vi "S4GUI.vi"(7 "Tab ObsEng":enum32{"Obs", "CCD modes", "Eng"}(tab)) -> ()   [LabVIEW 2018] (continued)
                n2773 = call "Write flatted cluster.vi"("error in (no error)"=w6126, "flatted cluster"=w6127, "Interface in"=w6081) -> ("error out"=w6123:errorcluster, "Interface out"=w6124:refnum<class "Interface.lvclass">)  [unwired: 7 in]
                n2774 = call-dynamic "Write Interface.vi"("error in (no error)"=w6123, "Interface.lvclass"=w6124, "Channel in"=w6076) -> ("error out"=w6121:errorcluster, "Channel out"=w6120:refnum<class "Channel.lvclass">)  [unwired: 7 in]
                n2775 = call "Write section_name.vi"("error in (no error)"=w6121, "section_name"="CCD_ACS4", "Channel in"=w6120) -> ("error out"=w6122:errorcluster, "Channel out"=w6117:refnum<class "Channel.lvclass">)  [unwired: 7 in]
                n2776 = call-dynamic "save config.vi"("error in (no error)"=w6122, "file config"="lastsaved.cfg", "Channel in"=w6117) -> ("error out"=w6099:errorcluster, "Channel out"=w6101:refnum<class "Channel.lvclass">)  [unwired: 7 in]
                n2777 = local read "Filter4"() -> (w6098:u8)
                n2778 = call-dynamic "Write Filter.vi"("error in (no error)"=w6099, "Filter"=w6098, "Channel in"=w6101) -> ("error out"=w6112:errorcluster, "Channel out"=w6100:refnum<class "Channel.lvclass">)  [unwired: 7 in]
                n2779 = call-dynamic "Read Interface.vi"("error in (no error)"=w6112, "Channel in"=w6100) -> ("error out"=w6111:errorcluster, "Interface.lvclass"=w6110:refnum<class "Interface.lvclass">, "Channel out"=w6052:refnum<class "Channel.lvclass">)  [unwired: 7 in]
                n2780 = call-dynamic "Write Suffix.vi"("error in (no error)"=w6111, "Suffix"=w6091, "Interface in"=w6110) -> ("error out"=w6102:errorcluster, "Interface out"=w6105:refnum<class "Interface.lvclass">)  [unwired: 7 in]
                n2781 = call-dynamic "Write ObsType.vi"("error in (no error)"=w6102, "ObsType"=w6090, "Interface in"=w6105) -> ("error out"=w6103:errorcluster, "Interface out"=w6106:refnum<class "Interface.lvclass">)  [unwired: 7 in]
                n2782 = call-dynamic "Write Object.vi"("error in (no error)"=w6103, "Object"=w6097, "Interface in"=w6106) -> ("error out"=w6104:errorcluster, "Interface out"=w6107:refnum<class "Interface.lvclass">)  [unwired: 7 in]
                n2783 = call-dynamic "Write Comments.vi"("error in (no error)"=w6104, "Comments"=w6096, "Interface in"=w6107) -> ("error out"=w6108:errorcluster, "Interface out"=w6109:refnum<class "Interface.lvclass">)  [unwired: 7 in]
                n2784 = call-dynamic "Write Observer.vi"("error in (no error)"=w6108, "Observer"=w6095, "Interface in"=w6109) -> ("error out"=w6050:errorcluster, "Interface out"=w6051:refnum<class "Interface.lvclass">)  [unwired: 7 in]
                n2785 = call-dynamic "Write Interface.vi"("error in (no error)"=w6050, "Interface.lvclass"=w6051, "Channel in"=w6052) -> ("error out"=w6059:errorcluster, "Channel out"=w6060:refnum<class "Channel.lvclass">)  [unwired: 7 in]
                n2786 = call-dynamic "Read State Machine.vi"("error in (no error)"=w6059, "Device in"=w6060) -> ("error out"=w6073:errorcluster, "State Machine.lvclass"=w6056:refnum<class "State Machine.lvclass">, "Device out"=w6061:refnum<class "Channel.lvclass">)  [unwired: 7 in]
                n2787 = call-dynamic "Read ref StatesQueue.vi"("error in (no error)"=w6073, "State Machine in"=w6056) -> ("error out"=w6071:errorcluster, "ref StatesQueue"=w6072:refnum<queue>, "State Machine out"=w6055:refnum<class "State Machine.lvclass">)  [unwired: 7 in]
                n2788 = Flush Queue(queue=w6072, error in (no error)=w6071) -> (queue out=w6070:refnum<queue>, error out=w6066:errorcluster)  [unwired: 1 out]
                n2789 = Enqueue Element(queue=w6070, element=u32 300 ("State"), error in (no error)=w6066) -> (queue out=w6069:refnum<queue>, error out=w6065:errorcluster)  [unwired: 1 in, 1 out]
                n2790 = Enqueue Element(queue=w6069, element=u32 60 ("State"), error in (no error)=w6065) -> (queue out=w6068:refnum<queue>, error out=w6067:errorcluster)  [unwired: 1 in, 1 out]
                n2791 = call-dynamic "Write ref StatesQueue.vi"("error in (no error)"=w6067, "ref StatesQueue"=w6068, "State Machine in"=w6055) -> ("error out"=w6064:errorcluster, "State Machine out"=w6054:refnum<class "State Machine.lvclass">)  [unwired: 7 in]
                n2792 = call-dynamic "Write State.vi"("error in (no error)"=w6064, "State"=0, "State Machine in"=w6054) -> ("error out"=w6075:errorcluster, "State Machine out"=w6053:refnum<class "State Machine.lvclass">)  [unwired: 7 in]
                n2793 = call-dynamic "Write State Machine.vi"("error in (no error)"=w6075, "State Machine.lvclass"=w6053, "Device in"=w6061) -> ("error out"=w6058:errorcluster, "Device out"=w6057:refnum<class "Channel.lvclass">)  [unwired: 7 in]
                n2794 = call-dynamic "Write Channel.vi"("error in (no error)"=w6058, "Channel.lvclass"=w6057, "Acquisition in"=w6130) -> ("error out"=w6113:errorcluster, "Acquisition out"=w6114:refnum<class "Acquisition.lvclass">)  [unwired: 7 in]
              }
            }
            n2795 = case shown="True" w6035 {
              tunnel: [w6327 w6406] -> w6046
              tunnel: [w6328 w6405] -> w6047
              tunnel: w6037 -> [w6328 w6388]
              tunnel: w6036 -> [w6327 w6387]
              tunnel: w6019 -> [_ w6366]
              tunnel: w6018 -> [_ w6365]
              tunnel: w6017 -> [_ w6364]
              tunnel: w6016 -> [_ w6360]
              tunnel: w6015 -> [_ w6359]
              frame False {
              }
              frame True {
                # "nome do arquivo .cfg"
                # "seção no arquivo .cfg"
                # "open"
                n2796 = call-dynamic "Read Channel.vi"("error in (no error)"=w6387, "Acquisition in"=w6388) -> ("error out"=w6407:errorcluster, "Channel.lvclass"=w6408:refnum<class "Channel.lvclass">, "Acquisition out"=w6409:refnum<class "Acquisition.lvclass">)  [unwired: 7 in]
                n2797 = call-dynamic "Read Interface.vi"("error in (no error)"=w6407, "Channel in"=w6408) -> ("error out"=w6357:errorcluster, "Interface.lvclass"=w6358:refnum<class "Interface.lvclass">, "Channel out"=w6347:refnum<class "Channel.lvclass">)  [unwired: 7 in]
                n2798 = call-dynamic "Read restoreExpTime.vi"("error in (no error)"=w6357, "Interface in"=w6358) -> ("error out"=w6355:errorcluster, "restoreExpTime"=w6354:bool, "Interface out"=w6356:refnum<class "Interface.lvclass">)  [unwired: 7 in]
                n2799 = case shown="True" w6354 {
                  tunnel: w6356 -> [w6411 w6416]
                  tunnel: [w6411 w6419] -> w6362
                  tunnel: w6355 -> [w6410 w6414]
                  tunnel: [w6410 w6418] -> w6361
                  frame False {
                  }
                  frame True {
                    n2800 = call-dynamic "Write restoreExpTime.vi"("error in (no error)"=w6414, "restoreExpTime"=FALSE, "Interface in"=w6416) -> ("error out"=w6413:errorcluster, "Interface out"=w6415:refnum<class "Interface.lvclass">)  [unwired: 7 in]
                    n2801 = call-dynamic "Read prev ExpTime.vi"("error in (no error)"=w6413, "Interface in"=w6415) -> ("error out"=w6418:errorcluster, "prev ExpTime"=w6417:dbl, "Interface out"=w6419:refnum<class "Interface.lvclass">)  [unwired: 7 in]
                    n2802 = property on="Exptime ch1" class="DigNum (strict)"("Value"=w6417) -> ()  [unwired: 2 in, 2 out]
                  }
                }
                n2803 = call-dynamic "Read PREV_FT.vi"("error in (no error)"=w6361, "Interface in"=w6362) -> ("error out"=w6353:errorcluster, "PREV_FT"=w6363:bool, "Interface out"=w6352:refnum<class "Interface.lvclass">)  [unwired: 7 in]
                n2804 = call-dynamic "Read target cluster.vi"("error in (no error)"=w6353, "Channel in"=w6347) -> ("error out"=w6348:errorcluster, "target cluster"=w6351:T30, "Channel out"=w6346:refnum<class "Channel.lvclass">)  [unwired: 7 in]
                n2805 = Bundle By Name(cluster=w6351, "SHUTTER_MODE"=u8 1, "FRAME_TRANSFER"=w6363) -> (w6350:T30)
                n2806 = call-dynamic "Write target cluster.vi"("error in (no error)"=w6348, "target cluster"=w6350, "Channel in"=w6346) -> ("error out"=w6349:errorcluster, "Channel out"=w6345:refnum<class "Channel.lvclass">)  [unwired: 7 in]
                n2807 = Flatten To String(anything=w6350, error in (no error)=w6349) -> (data string=w6404:string, error out=w6403:errorcluster)  [unwired: 2 in, 1 out]
                n2808 = call "Write flatted cluster.vi"("error in (no error)"=w6403, "flatted cluster"=w6404, "Interface in"=w6352) -> ("error out"=w6400:errorcluster, "Interface out"=w6401:refnum<class "Interface.lvclass">)  [unwired: 7 in]
                n2809 = call-dynamic "Write Interface.vi"("error in (no error)"=w6400, "Interface.lvclass"=w6401, "Channel in"=w6345) -> ("error out"=w6397:errorcluster, "Channel out"=w6396:refnum<class "Channel.lvclass">)  [unwired: 7 in]
                n2810 = call "Write section_name.vi"("error in (no error)"=w6397, "section_name"="CCD_ACS1", "Channel in"=w6396) -> ("error out"=w6398:errorcluster, "Channel out"=w6393:refnum<class "Channel.lvclass">)  [unwired: 7 in]
                n2811 = call-dynamic "save config.vi"("error in (no error)"=w6398, "file config"="lastsaved.cfg", "Channel in"=w6393) -> ("error out"=w6370:errorcluster, "Channel out"=w6369:refnum<class "Channel.lvclass">)  [unwired: 7 in]
                n2812 = local read "Filter1"() -> (w6371:u8)
                n2813 = call-dynamic "Write Filter.vi"("error in (no error)"=w6370, "Filter"=w6371, "Channel in"=w6369) -> ("error out"=w6386:errorcluster, "Channel out"=w6385:refnum<class "Channel.lvclass">)  [unwired: 7 in]
                n2814 = call-dynamic "Read Interface.vi"("error in (no error)"=w6386, "Channel in"=w6385) -> ("error out"=w6382:errorcluster, "Interface.lvclass"=w6381:refnum<class "Interface.lvclass">, "Channel out"=w6375:refnum<class "Channel.lvclass">)  [unwired: 7 in]
                n2815 = call-dynamic "Write Suffix.vi"("error in (no error)"=w6382, "Suffix"=w6360, "Interface in"=w6381) -> ("error out"=w6372:errorcluster, "Interface out"=w6376:refnum<class "Interface.lvclass">)  [unwired: 7 in]
                n2816 = call-dynamic "Write ObsType.vi"("error in (no error)"=w6372, "ObsType"=w6359, "Interface in"=w6376) -> ("error out"=w6373:errorcluster, "Interface out"=w6377:refnum<class "Interface.lvclass">)  [unwired: 7 in]
                n2817 = call-dynamic "Write Object.vi"("error in (no error)"=w6373, "Object"=w6366, "Interface in"=w6377) -> ("error out"=w6374:errorcluster, "Interface out"=w6378:refnum<class "Interface.lvclass">)  [unwired: 7 in]
                n2818 = call-dynamic "Write Comments.vi"("error in (no error)"=w6374, "Comments"=w6365, "Interface in"=w6378) -> ("error out"=w6379:errorcluster, "Interface out"=w6380:refnum<class "Interface.lvclass">)  [unwired: 7 in]
                n2819 = call-dynamic "Write Observer.vi"("error in (no error)"=w6379, "Observer"=w6364, "Interface in"=w6380) -> ("error out"=w6384:errorcluster, "Interface out"=w6383:refnum<class "Interface.lvclass">)  [unwired: 7 in]
                n2820 = call-dynamic "Write Interface.vi"("error in (no error)"=w6384, "Interface.lvclass"=w6383, "Channel in"=w6375) -> ("error out"=w6367:errorcluster, "Channel out"=w6368:refnum<class "Channel.lvclass">)  [unwired: 7 in]
                n2821 = call-dynamic "Read State Machine.vi"("error in (no error)"=w6367, "Device in"=w6368) -> ("error out"=w6342:errorcluster, "State Machine.lvclass"=w6343:refnum<class "State Machine.lvclass">, "Device out"=w6392:refnum<class "Channel.lvclass">)  [unwired: 7 in]
                n2822 = call-dynamic "Read ref StatesQueue.vi"("error in (no error)"=w6342, "State Machine in"=w6343) -> ("error out"=w6340:errorcluster, "ref StatesQueue"=w6341:refnum<queue>, "State Machine out"=w6336:refnum<class "State Machine.lvclass">)  [unwired: 7 in]
                n2823 = Flush Queue(queue=w6341, error in (no error)=w6340) -> (queue out=w6339:refnum<queue>, error out=w6334:errorcluster)  [unwired: 1 out]
                n2824 = Enqueue Element(queue=w6339, element=u32 300 ("State"), error in (no error)=w6334) -> (queue out=w6338:refnum<queue>, error out=w6333:errorcluster)  [unwired: 1 in, 1 out]
                n2825 = Enqueue Element(queue=w6338, element=u32 60 ("State"), error in (no error)=w6333) -> (queue out=w6337:refnum<queue>, error out=w6335:errorcluster)  [unwired: 1 in, 1 out]
                n2826 = call-dynamic "Write ref StatesQueue.vi"("error in (no error)"=w6335, "ref StatesQueue"=w6337, "State Machine in"=w6336) -> ("error out"=w6331:errorcluster, "State Machine out"=w6332:refnum<class "State Machine.lvclass">)  [unwired: 7 in]
                n2827 = call-dynamic "Write State.vi"("error in (no error)"=w6331, "State"=0, "State Machine in"=w6332) -> ("error out"=w6399:errorcluster, "State Machine out"=w6391:refnum<class "State Machine.lvclass">)  [unwired: 7 in]
                n2828 = call-dynamic "Write State Machine.vi"("error in (no error)"=w6399, "State Machine.lvclass"=w6391, "Device in"=w6392) -> ("error out"=w6389:errorcluster, "Device out"=w6390:refnum<class "Channel.lvclass">)  [unwired: 7 in]
                n2829 = call-dynamic "Write Channel.vi"("error in (no error)"=w6389, "Channel.lvclass"=w6390, "Acquisition in"=w6409) -> ("error out"=w6406:errorcluster, "Acquisition out"=w6405:refnum<class "Acquisition.lvclass">)  [unwired: 7 in]
              }
            }
            n2830 = case shown="True" w6032 {
              tunnel: w6034 -> [w6235 w6302]
              tunnel: w6033 -> [w6234 w6301]
              tunnel: [w6235 w6300] -> w6045
              tunnel: [w6234 w6299] -> w6044
              tunnel: w6019 -> [_ w6280]
              tunnel: w6018 -> [_ w6279]
              tunnel: w6017 -> [_ w6278]
              tunnel: w6016 -> [_ w6274]
              tunnel: w6015 -> [_ w6273]
              frame False {
              }
              frame True {
                # "nome do arquivo .cfg"
                # "seção no arquivo .cfg"
                # "open"
                n2831 = call-dynamic "Read Channel.vi"("error in (no error)"=w6301, "Acquisition in"=w6302) -> ("error out"=w6305:errorcluster, "Channel.lvclass"=w6304:refnum<class "Channel.lvclass">, "Acquisition out"=w6303:refnum<class "Acquisition.lvclass">)  [unwired: 7 in]
                n2832 = call-dynamic "Read Interface.vi"("error in (no error)"=w6305, "Channel in"=w6304) -> ("error out"=w6270:errorcluster, "Interface.lvclass"=w6272:refnum<class "Interface.lvclass">, "Channel out"=w6267:refnum<class "Channel.lvclass">)  [unwired: 7 in]
                n2833 = call-dynamic "Read restoreExpTime.vi"("error in (no error)"=w6270, "Interface in"=w6272) -> ("error out"=w6269:errorcluster, "restoreExpTime"=w6268:bool, "Interface out"=w6271:refnum<class "Interface.lvclass">)  [unwired: 7 in]
                n2834 = case shown="True" w6268 {
                  tunnel: w6271 -> [w6318 w6323]
                  tunnel: [w6318 w6326] -> w6276
                  tunnel: w6269 -> [w6317 w6322]
                  tunnel: [w6317 w6325] -> w6275
                  frame False {
                  }
                  frame True {
                    n2835 = call-dynamic "Write restoreExpTime.vi"("error in (no error)"=w6322, "restoreExpTime"=FALSE, "Interface in"=w6323) -> ("error out"=w6320:errorcluster, "Interface out"=w6321:refnum<class "Interface.lvclass">)  [unwired: 7 in]
                    n2836 = call-dynamic "Read prev ExpTime.vi"("error in (no error)"=w6320, "Interface in"=w6321) -> ("error out"=w6325:errorcluster, "prev ExpTime"=w6324:dbl, "Interface out"=w6326:refnum<class "Interface.lvclass">)  [unwired: 7 in]
                    n2837 = property on="Exptime ch2" class="DigNum (strict)"("Value"=w6324) -> ()  [unwired: 2 in, 2 out]
                  }
                }
                n2838 = call-dynamic "Read PREV_FT.vi"("error in (no error)"=w6275, "Interface in"=w6276) -> ("error out"=w6265:errorcluster, "PREV_FT"=w6277:bool, "Interface out"=w6264:refnum<class "Interface.lvclass">)  [unwired: 7 in]
                n2839 = call-dynamic "Read target cluster.vi"("error in (no error)"=w6265, "Channel in"=w6267) -> ("error out"=w6262:errorcluster, "target cluster"=w6266:T30, "Channel out"=w6260:refnum<class "Channel.lvclass">)  [unwired: 7 in]
                n2840 = Bundle By Name(cluster=w6266, "SHUTTER_MODE"=u8 1, "FRAME_TRANSFER"=w6277) -> (w6263:T30)
                n2841 = call-dynamic "Write target cluster.vi"("error in (no error)"=w6262, "target cluster"=w6263, "Channel in"=w6260) -> ("error out"=w6261:errorcluster, "Channel out"=w6259:refnum<class "Channel.lvclass">)  [unwired: 7 in]
                n2842 = Flatten To String(anything=w6263, error in (no error)=w6261) -> (data string=w6306:string, error out=w6307:errorcluster)  [unwired: 2 in, 1 out]
                n2843 = call "Write flatted cluster.vi"("error in (no error)"=w6307, "flatted cluster"=w6306, "Interface in"=w6264) -> ("error out"=w6310:errorcluster, "Interface out"=w6309:refnum<class "Interface.lvclass">)  [unwired: 7 in]
                n2844 = call-dynamic "Write Interface.vi"("error in (no error)"=w6310, "Interface.lvclass"=w6309, "Channel in"=w6259) -> ("error out"=w6312:errorcluster, "Channel out"=w6313:refnum<class "Channel.lvclass">)  [unwired: 7 in]
                n2845 = call "Write section_name.vi"("error in (no error)"=w6312, "section_name"="CCD_ACS2", "Channel in"=w6313) -> ("error out"=w6311:errorcluster, "Channel out"=w6316:refnum<class "Channel.lvclass">)  [unwired: 7 in]
                n2846 = call-dynamic "save config.vi"("error in (no error)"=w6311, "file config"="lastsaved.cfg", "Channel in"=w6316) -> ("error out"=w6282:errorcluster, "Channel out"=w6285:refnum<class "Channel.lvclass">)  [unwired: 7 in]
                n2847 = local read "Filter2"() -> (w6281:u8)
                n2848 = call-dynamic "Write Filter.vi"("error in (no error)"=w6282, "Filter"=w6281, "Channel in"=w6285) -> ("error out"=w6298:errorcluster, "Channel out"=w6284:refnum<class "Channel.lvclass">)  [unwired: 7 in]
                n2849 = call-dynamic "Read Interface.vi"("error in (no error)"=w6298, "Channel in"=w6284) -> ("error out"=w6295:errorcluster, "Interface.lvclass"=w6294:refnum<class "Interface.lvclass">, "Channel out"=w6283:refnum<class "Channel.lvclass">)  [unwired: 7 in]
                n2850 = call-dynamic "Write Suffix.vi"("error in (no error)"=w6295, "Suffix"=w6274, "Interface in"=w6294) -> ("error out"=w6286:errorcluster, "Interface out"=w6289:refnum<class "Interface.lvclass">)  [unwired: 7 in]
                n2851 = call-dynamic "Write ObsType.vi"("error in (no error)"=w6286, "ObsType"=w6273, "Interface in"=w6289) -> ("error out"=w6287:errorcluster, "Interface out"=w6290:refnum<class "Interface.lvclass">)  [unwired: 7 in]
                n2852 = call-dynamic "Write Object.vi"("error in (no error)"=w6287, "Object"=w6280, "Interface in"=w6290) -> ("error out"=w6288:errorcluster, "Interface out"=w6291:refnum<class "Interface.lvclass">)  [unwired: 7 in]
                n2853 = call-dynamic "Write Comments.vi"("error in (no error)"=w6288, "Comments"=w6279, "Interface in"=w6291) -> ("error out"=w6292:errorcluster, "Interface out"=w6293:refnum<class "Interface.lvclass">)  [unwired: 7 in]
                n2854 = call-dynamic "Write Observer.vi"("error in (no error)"=w6292, "Observer"=w6278, "Interface in"=w6293) -> ("error out"=w6297:errorcluster, "Interface out"=w6296:refnum<class "Interface.lvclass">)  [unwired: 7 in]
                n2855 = call-dynamic "Write Interface.vi"("error in (no error)"=w6297, "Interface.lvclass"=w6296, "Channel in"=w6283) -> ("error out"=w6237:errorcluster, "Channel out"=w6240:refnum<class "Channel.lvclass">)  [unwired: 7 in]
                n2856 = call-dynamic "Read State Machine.vi"("error in (no error)"=w6237, "Device in"=w6240) -> ("error out"=w6254:errorcluster, "State Machine.lvclass"=w6255:refnum<class "State Machine.lvclass">, "Device out"=w6239:refnum<class "Channel.lvclass">)  [unwired: 7 in]
                n2857 = call-dynamic "Read ref StatesQueue.vi"("error in (no error)"=w6254, "State Machine in"=w6255) -> ("error out"=w6252:errorcluster, "ref StatesQueue"=w6253:refnum<queue>, "State Machine out"=w6248:refnum<class "State Machine.lvclass">)  [unwired: 7 in]
                n2858 = Flush Queue(queue=w6253, error in (no error)=w6252) -> (queue out=w6251:refnum<queue>, error out=w6246:errorcluster)  [unwired: 1 out]
                n2859 = Enqueue Element(queue=w6251, element=u32 300 ("State"), error in (no error)=w6246) -> (queue out=w6250:refnum<queue>, error out=w6245:errorcluster)  [unwired: 1 in, 1 out]
                n2860 = Enqueue Element(queue=w6250, element=u32 60 ("State"), error in (no error)=w6245) -> (queue out=w6249:refnum<queue>, error out=w6247:errorcluster)  [unwired: 1 in, 1 out]
                n2861 = call-dynamic "Write ref StatesQueue.vi"("error in (no error)"=w6247, "ref StatesQueue"=w6249, "State Machine in"=w6248) -> ("error out"=w6243:errorcluster, "State Machine out"=w6244:refnum<class "State Machine.lvclass">)  [unwired: 7 in]
                n2862 = call-dynamic "Write State.vi"("error in (no error)"=w6243, "State"=0, "State Machine in"=w6244) -> ("error out"=w6258:errorcluster, "State Machine out"=w6257:refnum<class "State Machine.lvclass">)  [unwired: 7 in]
                n2863 = call-dynamic "Write State Machine.vi"("error in (no error)"=w6258, "State Machine.lvclass"=w6257, "Device in"=w6239) -> ("error out"=w6236:errorcluster, "Device out"=w6238:refnum<class "Channel.lvclass">)  [unwired: 7 in]
                n2864 = call-dynamic "Write Channel.vi"("error in (no error)"=w6236, "Channel.lvclass"=w6238, "Acquisition in"=w6303) -> ("error out"=w6299:errorcluster, "Acquisition out"=w6300:refnum<class "Acquisition.lvclass">)  [unwired: 7 in]
              }
            }
            n2865 = case shown="True" w6029 {
              tunnel: w6031 -> [w6142 w6209]
              tunnel: w6030 -> [w6141 w6208]
              tunnel: [w6142 w6207] -> w6043
              tunnel: [w6141 w6206] -> w6042
              tunnel: w6019 -> [_ w6187]
              tunnel: w6018 -> [_ w6186]
              tunnel: w6017 -> [_ w6185]
              tunnel: w6016 -> [_ w6181]
              tunnel: w6015 -> [_ w6180]
              frame False {
              }
              frame True {
                # "nome do arquivo .cfg"
                # "seção no arquivo .cfg"
                # "open"
                n2866 = call-dynamic "Read Channel.vi"("error in (no error)"=w6208, "Acquisition in"=w6209) -> ("error out"=w6212:errorcluster, "Channel.lvclass"=w6211:refnum<class "Channel.lvclass">, "Acquisition out"=w6210:refnum<class "Acquisition.lvclass">)  [unwired: 7 in]
                n2867 = call-dynamic "Read Interface.vi"("error in (no error)"=w6212, "Channel in"=w6211) -> ("error out"=w6177:errorcluster, "Interface.lvclass"=w6179:refnum<class "Interface.lvclass">, "Channel out"=w6174:refnum<class "Channel.lvclass">)  [unwired: 7 in]
                n2868 = call-dynamic "Read restoreExpTime.vi"("error in (no error)"=w6177, "Interface in"=w6179) -> ("error out"=w6176:errorcluster, "restoreExpTime"=w6175:bool, "Interface out"=w6178:refnum<class "Interface.lvclass">)  [unwired: 7 in]
                n2869 = case shown="True" w6175 {
                  tunnel: w6178 -> [w6225 w6230]
                  tunnel: [w6225 w6233] -> w6183
                  tunnel: w6176 -> [w6224 w6229]
                  tunnel: [w6224 w6232] -> w6182
                  frame False {
                  }
                  frame True {
                    n2870 = call-dynamic "Write restoreExpTime.vi"("error in (no error)"=w6229, "restoreExpTime"=FALSE, "Interface in"=w6230) -> ("error out"=w6227:errorcluster, "Interface out"=w6228:refnum<class "Interface.lvclass">)  [unwired: 7 in]
                    n2871 = call-dynamic "Read prev ExpTime.vi"("error in (no error)"=w6227, "Interface in"=w6228) -> ("error out"=w6232:errorcluster, "prev ExpTime"=w6231:dbl, "Interface out"=w6233:refnum<class "Interface.lvclass">)  [unwired: 7 in]
                    n2872 = property on="Exptime ch3" class="DigNum (strict)"("Value"=w6231) -> ()  [unwired: 2 in, 2 out]
                  }
                }
                n2873 = call-dynamic "Read PREV_FT.vi"("error in (no error)"=w6182, "Interface in"=w6183) -> ("error out"=w6172:errorcluster, "PREV_FT"=w6184:bool, "Interface out"=w6171:refnum<class "Interface.lvclass">)  [unwired: 7 in]
                n2874 = call-dynamic "Read target cluster.vi"("error in (no error)"=w6172, "Channel in"=w6174) -> ("error out"=w6169:errorcluster, "target cluster"=w6173:T30, "Channel out"=w6167:refnum<class "Channel.lvclass">)  [unwired: 7 in]
                n2875 = Bundle By Name(cluster=w6173, "SHUTTER_MODE"=u8 1, "FRAME_TRANSFER"=w6184) -> (w6170:T30)
                n2876 = call-dynamic "Write target cluster.vi"("error in (no error)"=w6169, "target cluster"=w6170, "Channel in"=w6167) -> ("error out"=w6168:errorcluster, "Channel out"=w6166:refnum<class "Channel.lvclass">)  [unwired: 7 in]
                n2877 = Flatten To String(anything=w6170, error in (no error)=w6168) -> (data string=w6213:string, error out=w6214:errorcluster)  [unwired: 2 in, 1 out]
                n2878 = call "Write flatted cluster.vi"("error in (no error)"=w6214, "flatted cluster"=w6213, "Interface in"=w6171) -> ("error out"=w6217:errorcluster, "Interface out"=w6216:refnum<class "Interface.lvclass">)  [unwired: 7 in]
                n2879 = call-dynamic "Write Interface.vi"("error in (no error)"=w6217, "Interface.lvclass"=w6216, "Channel in"=w6166) -> ("error out"=w6219:errorcluster, "Channel out"=w6220:refnum<class "Channel.lvclass">)  [unwired: 7 in]
                n2880 = call "Write section_name.vi"("error in (no error)"=w6219, "section_name"="CCD_ACS3", "Channel in"=w6220) -> ("error out"=w6218:errorcluster, "Channel out"=w6223:refnum<class "Channel.lvclass">)  [unwired: 7 in]
                n2881 = call-dynamic "save config.vi"("error in (no error)"=w6218, "file config"="lastsaved.cfg", "Channel in"=w6223) -> ("error out"=w6189:errorcluster, "Channel out"=w6190:refnum<class "Channel.lvclass">)  [unwired: 7 in]
                n2882 = local read "Filter3"() -> (w6188:u8)
                n2883 = call-dynamic "Write Filter.vi"("error in (no error)"=w6189, "Filter"=w6188, "Channel in"=w6190) -> ("error out"=w6191:errorcluster, "Channel out"=w6204:refnum<class "Channel.lvclass">)  [unwired: 7 in]
                n2884 = call-dynamic "Read Interface.vi"("error in (no error)"=w6191, "Channel in"=w6204) -> ("error out"=w6194:errorcluster, "Interface.lvclass"=w6195:refnum<class "Interface.lvclass">, "Channel out"=w6205:refnum<class "Channel.lvclass">)  [unwired: 7 in]
                n2885 = call-dynamic "Write Suffix.vi"("error in (no error)"=w6194, "Suffix"=w6181, "Interface in"=w6195) -> ("error out"=w6203:errorcluster, "Interface out"=w6200:refnum<class "Interface.lvclass">)  [unwired: 7 in]
                n2886 = call-dynamic "Write ObsType.vi"("error in (no error)"=w6203, "ObsType"=w6180, "Interface in"=w6200) -> ("error out"=w6202:errorcluster, "Interface out"=w6199:refnum<class "Interface.lvclass">)  [unwired: 7 in]
                n2887 = call-dynamic "Write Object.vi"("error in (no error)"=w6202, "Object"=w6187, "Interface in"=w6199) -> ("error out"=w6201:errorcluster, "Interface out"=w6198:refnum<class "Interface.lvclass">)  [unwired: 7 in]
                n2888 = call-dynamic "Write Comments.vi"("error in (no error)"=w6201, "Comments"=w6186, "Interface in"=w6198) -> ("error out"=w6197:errorcluster, "Interface out"=w6196:refnum<class "Interface.lvclass">)  [unwired: 7 in]
                n2889 = call-dynamic "Write Observer.vi"("error in (no error)"=w6197, "Observer"=w6185, "Interface in"=w6196) -> ("error out"=w6192:errorcluster, "Interface out"=w6193:refnum<class "Interface.lvclass">)  [unwired: 7 in]
                n2890 = call-dynamic "Write Interface.vi"("error in (no error)"=w6192, "Interface.lvclass"=w6193, "Channel in"=w6205) -> ("error out"=w6145:errorcluster, "Channel out"=w6146:refnum<class "Channel.lvclass">)  [unwired: 7 in]
                n2891 = call-dynamic "Read State Machine.vi"("error in (no error)"=w6145, "Device in"=w6146) -> ("error out"=w6161:errorcluster, "State Machine.lvclass"=w6162:refnum<class "State Machine.lvclass">, "Device out"=w6147:refnum<class "Channel.lvclass">)  [unwired: 7 in]
                n2892 = call-dynamic "Read ref StatesQueue.vi"("error in (no error)"=w6161, "State Machine in"=w6162) -> ("error out"=w6159:errorcluster, "ref StatesQueue"=w6160:refnum<queue>, "State Machine out"=w6155:refnum<class "State Machine.lvclass">)  [unwired: 7 in]
                n2893 = Flush Queue(queue=w6160, error in (no error)=w6159) -> (queue out=w6158:refnum<queue>, error out=w6153:errorcluster)  [unwired: 1 out]
                n2894 = Enqueue Element(queue=w6158, element=u32 300 ("State"), error in (no error)=w6153) -> (queue out=w6157:refnum<queue>, error out=w6152:errorcluster)  [unwired: 1 in, 1 out]
                n2895 = Enqueue Element(queue=w6157, element=u32 60 ("State"), error in (no error)=w6152) -> (queue out=w6156:refnum<queue>, error out=w6154:errorcluster)  [unwired: 1 in, 1 out]
                n2896 = call-dynamic "Write ref StatesQueue.vi"("error in (no error)"=w6154, "ref StatesQueue"=w6156, "State Machine in"=w6155) -> ("error out"=w6150:errorcluster, "State Machine out"=w6151:refnum<class "State Machine.lvclass">)  [unwired: 7 in]
                n2897 = call-dynamic "Write State.vi"("error in (no error)"=w6150, "State"=0, "State Machine in"=w6151) -> ("error out"=w6165:errorcluster, "State Machine out"=w6164:refnum<class "State Machine.lvclass">)  [unwired: 7 in]
                n2898 = call-dynamic "Write State Machine.vi"("error in (no error)"=w6165, "State Machine.lvclass"=w6164, "Device in"=w6147) -> ("error out"=w6144:errorcluster, "Device out"=w6143:refnum<class "Channel.lvclass">)  [unwired: 7 in]
                n2899 = call-dynamic "Write Channel.vi"("error in (no error)"=w6144, "Channel.lvclass"=w6143, "Acquisition in"=w6210) -> ("error out"=w6206:errorcluster, "Acquisition out"=w6207:refnum<class "Acquisition.lvclass">)  [unwired: 7 in]
              }
            }
          }
        }
        n2900 = call-dynamic "Write AcquisitionA.vi"("error in (no error)"=w5166, "Acquisition.lvclass"=w5167, "S4ACS_GUI in"=w5168) -> ("error out"=w5158:errorcluster, "S4ACS_GUI out"=w5162:refnum<class "S4GUI.lvclass">)  [unwired: 7 in]
        n2901 = call "Write AcquisitionB.vi"("error in (no error)"=w5163, "Acquisition.lvclass"=w5164, "S4ACS_GUI in"=w5162) -> ("error out"=w5157:errorcluster, "S4ACS_GUI out"=w5161:refnum<class "S4GUI.lvclass">)  [unwired: 7 in]
        n2902 = call-dynamic "Write AcquisitionC.vi"("error in (no error)"=w5152, "Acquisition.lvclass"=w5153, "S4ACS_GUI in"=w5161) -> ("error out"=w5156:errorcluster, "S4ACS_GUI out"=w5160:refnum<class "S4GUI.lvclass">)  [unwired: 7 in]
        n2903 = call-dynamic "Write AcquisitionD.vi"("error in (no error)"=w5150, "Acquisition.lvclass"=w5151, "S4ACS_GUI in"=w5160) -> ("error out"=w5155:errorcluster, "S4ACS_GUI out"=w5159:refnum<class "S4GUI.lvclass">)  [unwired: 7 in]
        n2904 = Merge Errors(w5158, w5157, w5156, w5155) -> (w5154:errorcluster)
        n2905 = call "Write cfg file.vi"("error in (no error)"=w5154, "cfg file"="lastsaved.cfg", "S4ACS_GUI in"=w5159) -> ("error out"=w5108:errorcluster, "S4ACS_GUI out"=w5109:refnum<class "S4GUI.lvclass">)  [unwired: 7 in]
        n2906 = disable-structure shown="Enabled" {
          disable-tunnel: w5109 -> [w5172 w5207]
          disable-tunnel: w5108 -> [w5171 w5206]
          disable-tunnel: [w5170 w5207] -> w5107
          disable-tunnel: [w5169 w5206] -> w5106
          frame Disabled {
            # "Este código passou para o evento \"Timeout\" (executa sempre)"
            # "1a vez FOTOM (F)"
            # "1a vez POLAR (F)"
            n2907 = call "Read Instrument.lvclass.vi"("error in (no error)"=w5171, "S4ACS_GUI in"=w5172) -> ("error out"=w5174:errorcluster, "Instrument.lvclass"=w5175:refnum<class "Instrument.lvclass">, "S4ACS_GUI out"=w5170:refnum<class "S4GUI.lvclass">)  [unwired: 7 in]
            n2908 = call-dynamic "Read mode.vi"("error in (no error)"=w5174, "Instrument in"=w5175) -> ("error out"=w5169:errorcluster, "mode"=w5173:bool)  [unwired: 7 in, 1 out]
            n2909 = while {
              tunnel: w5173 -> [w5180]
              shift-right: [w5176] -> _
              shift-left: _ -> [w5179]
              shift-right: [w5177] -> _
              shift-left: _ -> [w5178]
              stop <- TRUE stop-if-true
              # "Valores default para procedimento\nde ajuste de foco do telescópio"
              n2910 = case shown="True" w5180 {
                tunnel: w5179 -> [w5182 w5197]
                tunnel: [w5183 w5196] -> w5176
                tunnel: w5178 -> [w5185 w5195]
                tunnel: [w5184 w5194] -> w5177
                frame True {
                  # "polarimetria"
                  n2911 = case shown="False" w5185 {
                    selector: w5185 -> [w5189 w5193]
                    tunnel: [w5188 w5193] -> w5184
                    tunnel: [FALSE FALSE] -> w5183
                    tunnel: w5182 -> [_ _]
                    frame False {
                      w5186 = 12900
                      n2912 = local write "Start focus"(w5186) -> ()
                      n2913 = local write "Target focus"(w5186) -> ()
                      n2914 = local write "Step focus"(80) -> ()
                      n2915 = local write "#steps"(11) -> ()
                      n2916 = Not(x=w5189) -> (.not. x?=w5188:bool)
                    }
                    frame True {
                    }
                  }
                }
                frame False {
                  # "fotometria"
                  n2917 = case shown="False" w5197 {
                    selector: w5197 -> [w5200 w5205]
                    tunnel: [w5199 w5205] -> w5196
                    tunnel: w5195 -> [_ _]
                    tunnel: [FALSE FALSE] -> w5194
                    frame False {
                      w5198 = 13400
                      n2918 = local write "Start focus"(w5198) -> ()
                      n2919 = local write "Step focus"(100) -> ()
                      n2920 = local write "Target focus"(w5198) -> ()
                      n2921 = local write "#steps"(11) -> ()
                      n2922 = Not(x=w5200) -> (.not. x?=w5199:bool)
                    }
                    frame True {
                    }
                  }
                }
              }
            }
          }
          frame Enabled {
          }
        }
      }
      event "set keywords", "set Observer": Value Change {
        # "SET Observer, suffix, comments e object da aba selecionada."
        n2923 = event-data() -> ()  [unwired: 1 in, 1 out]
        n2924 = local read "Tab Acq Type"() -> (w6458:T1)
        n2925 = case shown="\"DFLAT\"" w6458 {
          tunnel: ["OBJECT" "FLAT" "FLAT" "DARK" "ZERO" "FOCUS"] -> w6433
          tunnel: [w6663 w6667 w6671 w6675 w6679 w6684] -> w6434
          tunnel: [w6662 w6666 w6670 w6674 w6678 w6683] -> w6428
          tunnel: [w6661 w6665 w6669 w6673 w6677 w6682] -> w6427
          tunnel: [_ _ _ _ _ TRUE] -> _
          frame "OBJECT", Default {
            n2926 = local read "OBJECT Comments"() -> (w6661:string)
            n2927 = local read "Object_obj"() -> (w6663:string)
            n2928 = local read "object suffix"() -> (w6662:string)
          }
          frame "DFLAT" {
            n2929 = local read "DFLAT Comments"() -> (w6665:string)
            n2930 = local read "Object_dflat"() -> (w6667:string)
            n2931 = local read "dflat suffix"() -> (w6666:string)
          }
          frame "SFLAT" {
            n2932 = local read "SFLAT Comments"() -> (w6669:string)
            n2933 = local read "Object_sflat"() -> (w6671:string)
            n2934 = local read "sflat suffix"() -> (w6670:string)
          }
          frame "DARK" {
            n2935 = local read "DARK Comments"() -> (w6673:string)
            n2936 = local read "Object_dark"() -> (w6675:string)
            n2937 = local read "dark suffix"() -> (w6674:string)
          }
          frame "ZERO" {
            n2938 = local read "ZERO Comments"() -> (w6677:string)
            n2939 = local read "Object_zero"() -> (w6679:string)
            n2940 = local read "zero suffix"() -> (w6678:string)
          }
          frame "FOCUS" {
            n2941 = local read "FOCUS Comments"() -> (w6682:string)
            n2942 = local read "Object_focus"() -> (w6684:string)
            n2943 = local read "focus suffix"() -> (w6683:string)
          }
        }
        n2944 = call-dynamic "Write User Event.vi"("error in (no error)"=w6422, "User Event"="SET KEYWORDS CLICKED (Obsever, ProjectID, Object, Comments) ", "S4GUI in"=w6423) -> ("error out"=w6420:errorcluster, "S4GUI out"=w6421:refnum<class "S4GUI.lvclass">)  [unwired: 7 in]
        n2945 = call-dynamic "Read Publisher.lvclass.vi"("error in (no error)"=w6420, "S4GUI in"=w6421) -> ("error out"=w6444:errorcluster, "Publisher.lvclass"=w6440:refnum<class "Publisher.lvclass">, "S4GUI out"=w6445:refnum<class "S4GUI.lvclass">)  [unwired: 7 in]
        n2946 = call-dynamic "Write object.vi"("error in (no error)"=w6444, "object"=w6434, "Publisher in"=w6440) -> ("error out"=w6443:errorcluster, "Publisher out"=w6439:refnum<class "Publisher.lvclass">)  [unwired: 7 in]
        n2947 = call-dynamic "Write obstype.vi"("error in (no error)"=w6443, "obstype"=w6433, "Publisher in"=w6439) -> ("error out"=w6442:errorcluster, "Publisher out"=w6438:refnum<class "Publisher.lvclass">)  [unwired: 7 in]
        n2948 = call-dynamic "Write observer.vi"("error in (no error)"=w6442, "observer"=w6432, "Publisher in"=w6438) -> ("error out"=w6441:errorcluster, "Publisher out"=w6437:refnum<class "Publisher.lvclass">)  [unwired: 7 in]
        n2949 = call-dynamic "Write projid.vi"("error in (no error)"=w6441, "projid"=w6431, "Publisher in"=w6437) -> ("error out"=w6426:errorcluster, "Publisher out"=w6425:refnum<class "Publisher.lvclass">)  [unwired: 7 in]
        n2950 = call-dynamic "Write comments.vi"("error in (no error)"=w6426, "comments"=w6427, "Publisher in"=w6425) -> ("error out"=w6430:errorcluster, "Publisher out"=w6429:refnum<class "Publisher.lvclass">)  [unwired: 7 in]
        n2951 = call-dynamic "Write Publisher.lvclass.vi"("error in (no error)"=w6430, "Publisher.lvclass"=w6429, "S4GUI in"=w6445) -> ("error out"=w6435:errorcluster, "S4GUI out"=w6436:refnum<class "S4GUI.lvclass">)  [unwired: 7 in]
        n2952 = call-dynamic "Read AcquisitionC.vi"("error in (no error)"=w6435, "S4ACS_GUI in"=w6436) -> ("error out"=w6462:errorcluster, "Acquisition.lvclass"=w6463:refnum<class "Acquisition.lvclass">)  [unwired: 7 in, 1 out]
        n2953 = call-dynamic "Read AcquisitionA.vi"("error in (no error)"=w6435, "S4ACS_GUI in"=w6436) -> ("error out"=w6466:errorcluster, "Acquisition.lvclass"=w6467:refnum<class "Acquisition.lvclass">, "S4ACS_GUI out"=w6488:refnum<class "S4GUI.lvclass">)  [unwired: 7 in]
        n2954 = call "Read AcquisitionB.vi"("error in (no error)"=w6435, "S4ACS_GUI in"=w6436) -> ("error out"=w6464:errorcluster, "Acquisition.lvclass"=w6465:refnum<class "Acquisition.lvclass">)  [unwired: 7 in, 1 out]
        n2955 = call-dynamic "Read AcquisitionD.vi"("error in (no error)"=w6435, "S4ACS_GUI in"=w6436) -> ("error out"=w6460:errorcluster, "Acquisition.lvclass"=w6461:refnum<class "Acquisition.lvclass">)  [unwired: 7 in, 1 out]
        n2956 = call-dynamic "Read enabled.vi"("error in (no error)"=w6460, "Server in"=w6461) -> ("error out"=w6447:errorcluster, "enabled"=w6446:bool, "Server out"=w6448:refnum<class "Acquisition.lvclass">)  [unwired: 7 in]
        n2957 = call-dynamic "Read enabled.vi"("error in (no error)"=w6462, "Server in"=w6463) -> ("error out"=w6450:errorcluster, "enabled"=w6449:bool, "Server out"=w6451:refnum<class "Acquisition.lvclass">)  [unwired: 7 in]
        n2958 = call-dynamic "Read enabled.vi"("error in (no error)"=w6464, "Server in"=w6465) -> ("error out"=w6453:errorcluster, "enabled"=w6452:bool, "Server out"=w6454:refnum<class "Acquisition.lvclass">)  [unwired: 7 in]
        n2959 = call-dynamic "Read enabled.vi"("error in (no error)"=w6466, "Server in"=w6467) -> ("error out"=w6456:errorcluster, "enabled"=w6455:bool, "Server out"=w6457:refnum<class "Acquisition.lvclass">)  [unwired: 7 in]
        n2960 = To Lower Case(string=w6428) -> (all lower case string=w6459:string)
        n2961 = case shown="True" w6452 {
          tunnel: w6454 -> [w6576 w6608]
          tunnel: w6453 -> [w6575 w6607]
          tunnel: [w6576 w6606] -> w6482
          tunnel: [w6575 w6605] -> w6481
          tunnel: w6459 -> [_ w6588]
          tunnel: w6433 -> [_ w6587]
          tunnel: w6434 -> [_ w6586]
          tunnel: w6427 -> [_ w6585]
          tunnel: w6432 -> [_ w6584]
          tunnel: w6431 -> [_ w6579]
          frame False {
          }
          frame True {
            (unwired) 12 ("State")
            n2962 = call-dynamic "Read Channel.vi"("error in (no error)"=w6607, "Acquisition in"=w6608) -> ("error out"=w6582:errorcluster, "Channel.lvclass"=w6583:refnum<class "Channel.lvclass">, "Acquisition out"=w6609:refnum<class "Acquisition.lvclass">)  [unwired: 7 in]
            n2963 = local read "Filter2"() -> (w6589:u8)
            n2964 = call-dynamic "Write Filter.vi"("error in (no error)"=w6582, "Filter"=w6589, "Channel in"=w6583) -> ("error out"=w6604:errorcluster, "Channel out"=w6593:refnum<class "Channel.lvclass">)  [unwired: 7 in]
            n2965 = call-dynamic "Read Interface.vi"("error in (no error)"=w6604, "Channel in"=w6593) -> ("error out"=w6603:errorcluster, "Interface.lvclass"=w6602:refnum<class "Interface.lvclass">, "Channel out"=w6592:refnum<class "Channel.lvclass">)  [unwired: 7 in]
            n2966 = call-dynamic "Write Suffix.vi"("error in (no error)"=w6603, "Suffix"=w6588, "Interface in"=w6602) -> ("error out"=w6594:errorcluster, "Interface out"=w6597:refnum<class "Interface.lvclass">)  [unwired: 7 in]
            n2967 = call-dynamic "Write ObsType.vi"("error in (no error)"=w6594, "ObsType"=w6587, "Interface in"=w6597) -> ("error out"=w6595:errorcluster, "Interface out"=w6598:refnum<class "Interface.lvclass">)  [unwired: 7 in]
            n2968 = call-dynamic "Write Object.vi"("error in (no error)"=w6595, "Object"=w6586, "Interface in"=w6598) -> ("error out"=w6596:errorcluster, "Interface out"=w6599:refnum<class "Interface.lvclass">)  [unwired: 7 in]
            n2969 = call-dynamic "Write Comments.vi"("error in (no error)"=w6596, "Comments"=w6585, "Interface in"=w6599) -> ("error out"=w6600:errorcluster, "Interface out"=w6601:refnum<class "Interface.lvclass">)  [unwired: 7 in]
            n2970 = call-dynamic "Write Observer.vi"("error in (no error)"=w6600, "Observer"=w6584, "Interface in"=w6601) -> ("error out"=w6581:errorcluster, "Interface out"=w6580:refnum<class "Interface.lvclass">)  [unwired: 7 in]
            n2971 = call-dynamic "Write Project ID.vi"("error in (no error)"=w6581, "Project ID"=w6579, "Interface in"=w6580) -> ("error out"=w6577:errorcluster, "Interface out"=w6578:refnum<class "Interface.lvclass">)  [unwired: 7 in]
            n2972 = call-dynamic "Write Interface.vi"("error in (no error)"=w6577, "Interface.lvclass"=w6578, "Channel in"=w6592) -> ("error out"=w6590:errorcluster, "Channel out"=w6591:refnum<class "Channel.lvclass">)  [unwired: 7 in]
            n2973 = call-dynamic "Read State Machine.vi"("error in (no error)"=w6590, "Device in"=w6591) -> ("error out"=w6610:errorcluster, "State Machine.lvclass"=w6614:refnum<class "State Machine.lvclass">, "Device out"=w6613:refnum<class "Channel.lvclass">)  [unwired: 7 in]
            n2974 = call-dynamic "Write State.vi"("error in (no error)"=w6610, "State"=300, "State Machine in"=w6614) -> ("error out"=w6611:errorcluster, "State Machine out"=w6615:refnum<class "State Machine.lvclass">)  [unwired: 7 in]
            n2975 = call-dynamic "Write State Machine.vi"("error in (no error)"=w6611, "State Machine.lvclass"=w6615, "Device in"=w6613) -> ("error out"=w6617:errorcluster, "Device out"=w6616:refnum<class "Channel.lvclass">)  [unwired: 7 in]
            n2976 = call-dynamic "Write Channel.vi"("error in (no error)"=w6617, "Channel.lvclass"=w6616, "Acquisition in"=w6609) -> ("error out"=w6605:errorcluster, "Acquisition out"=w6606:refnum<class "Acquisition.lvclass">)  [unwired: 7 in]
          }
        }
        n2977 = case shown="True" w6455 {
          tunnel: [w6618 w6659] -> w6486
          tunnel: [w6619 w6658] -> w6487
          tunnel: w6457 -> [w6619 w6649]
          tunnel: w6456 -> [w6618 w6648]
          tunnel: w6459 -> [_ w6631]
          tunnel: w6433 -> [_ w6630]
          tunnel: w6434 -> [_ w6629]
          tunnel: w6427 -> [_ w6628]
          tunnel: w6432 -> [_ w6627]
          tunnel: w6431 -> [_ w6624]
          frame False {
          }
          frame True {
            (unwired) 12 ("State")
            n2978 = call-dynamic "Read Channel.vi"("error in (no error)"=w6648, "Acquisition in"=w6649) -> ("error out"=w6625:errorcluster, "Channel.lvclass"=w6626:refnum<class "Channel.lvclass">, "Acquisition out"=w6660:refnum<class "Acquisition.lvclass">)  [unwired: 7 in]
            n2979 = local read "Filter1"() -> (w6634:u8)
            n2980 = call-dynamic "Write Filter.vi"("error in (no error)"=w6625, "Filter"=w6634, "Channel in"=w6626) -> ("error out"=w6647:errorcluster, "Channel out"=w6646:refnum<class "Channel.lvclass">)  [unwired: 7 in]
            n2981 = call-dynamic "Read Interface.vi"("error in (no error)"=w6647, "Channel in"=w6646) -> ("error out"=w6645:errorcluster, "Interface.lvclass"=w6644:refnum<class "Interface.lvclass">, "Channel out"=w6638:refnum<class "Channel.lvclass">)  [unwired: 7 in]
            n2982 = call-dynamic "Write Suffix.vi"("error in (no error)"=w6645, "Suffix"=w6631, "Interface in"=w6644) -> ("error out"=w6635:errorcluster, "Interface out"=w6639:refnum<class "Interface.lvclass">)  [unwired: 7 in]
            n2983 = call-dynamic "Write ObsType.vi"("error in (no error)"=w6635, "ObsType"=w6630, "Interface in"=w6639) -> ("error out"=w6636:errorcluster, "Interface out"=w6640:refnum<class "Interface.lvclass">)  [unwired: 7 in]
            n2984 = call-dynamic "Write Object.vi"("error in (no error)"=w6636, "Object"=w6629, "Interface in"=w6640) -> ("error out"=w6637:errorcluster, "Interface out"=w6641:refnum<class "Interface.lvclass">)  [unwired: 7 in]
            n2985 = call-dynamic "Write Comments.vi"("error in (no error)"=w6637, "Comments"=w6628, "Interface in"=w6641) -> ("error out"=w6642:errorcluster, "Interface out"=w6643:refnum<class "Interface.lvclass">)  [unwired: 7 in]
            n2986 = call-dynamic "Write Observer.vi"("error in (no error)"=w6642, "Observer"=w6627, "Interface in"=w6643) -> ("error out"=w6622:errorcluster, "Interface out"=w6623:refnum<class "Interface.lvclass">)  [unwired: 7 in]
            n2987 = call-dynamic "Write Project ID.vi"("error in (no error)"=w6622, "Project ID"=w6624, "Interface in"=w6623) -> ("error out"=w6620:errorcluster, "Interface out"=w6621:refnum<class "Interface.lvclass">)  [unwired: 7 in]
            n2988 = call-dynamic "Write Interface.vi"("error in (no error)"=w6620, "Interface.lvclass"=w6621, "Channel in"=w6638) -> ("error out"=w6632:errorcluster, "Channel out"=w6633:refnum<class "Channel.lvclass">)  [unwired: 7 in]
            n2989 = call-dynamic "Read State Machine.vi"("error in (no error)"=w6632, "Device in"=w6633) -> ("error out"=w6657:errorcluster, "State Machine.lvclass"=w6653:refnum<class "State Machine.lvclass">, "Device out"=w6654:refnum<class "Channel.lvclass">)  [unwired: 7 in]
            n2990 = call-dynamic "Write State.vi"("error in (no error)"=w6657, "State"=300, "State Machine in"=w6653) -> ("error out"=w6656:errorcluster, "State Machine out"=w6652:refnum<class "State Machine.lvclass">)  [unwired: 7 in]
            n2991 = call-dynamic "Write State Machine.vi"("error in (no error)"=w6656, "State Machine.lvclass"=w6652, "Device in"=w6654) -> ("error out"=w6650:errorcluster, "Device out"=w6651:refnum<class "Channel.lvclass">)  [unwired: 7 in]
            n2992 = call-dynamic "Write Channel.vi"("error in (no error)"=w6650, "Channel.lvclass"=w6651, "Acquisition in"=w6660) -> ("error out"=w6659:errorcluster, "Acquisition out"=w6658:refnum<class "Acquisition.lvclass">)  [unwired: 7 in]
          }
        }
        n2993 = case shown="True" w6449 {
          tunnel: w6451 -> [w6533 w6565]
          tunnel: w6450 -> [w6532 w6564]
          tunnel: [w6533 w6563] -> w6471
          tunnel: [w6532 w6562] -> w6470
          tunnel: w6459 -> [_ w6545]
          tunnel: w6433 -> [_ w6544]
          tunnel: w6434 -> [_ w6543]
          tunnel: w6427 -> [_ w6542]
          tunnel: w6432 -> [_ w6541]
          tunnel: w6431 -> [_ w6536]
          frame False {
          }
          frame True {
            (unwired) 12 ("State")
            n2994 = call-dynamic "Read Channel.vi"("error in (no error)"=w6564, "Acquisition in"=w6565) -> ("error out"=w6539:errorcluster, "Channel.lvclass"=w6540:refnum<class "Channel.lvclass">, "Acquisition out"=w6566:refnum<class "Acquisition.lvclass">)  [unwired: 7 in]
            n2995 = local read "Filter3"() -> (w6546:u8)
            n2996 = call-dynamic "Write Filter.vi"("error in (no error)"=w6539, "Filter"=w6546, "Channel in"=w6540) -> ("error out"=w6549:errorcluster, "Channel out"=w6560:refnum<class "Channel.lvclass">)  [unwired: 7 in]
            n2997 = call-dynamic "Read Interface.vi"("error in (no error)"=w6549, "Channel in"=w6560) -> ("error out"=w6550:errorcluster, "Interface.lvclass"=w6551:refnum<class "Interface.lvclass">, "Channel out"=w6561:refnum<class "Channel.lvclass">)  [unwired: 7 in]
            n2998 = call-dynamic "Write Suffix.vi"("error in (no error)"=w6550, "Suffix"=w6545, "Interface in"=w6551) -> ("error out"=w6559:errorcluster, "Interface out"=w6556:refnum<class "Interface.lvclass">)  [unwired: 7 in]
            n2999 = call-dynamic "Write ObsType.vi"("error in (no error)"=w6559, "ObsType"=w6544, "Interface in"=w6556) -> ("error out"=w6558:errorcluster, "Interface out"=w6555:refnum<class "Interface.lvclass">)  [unwired: 7 in]
            n3000 = call-dynamic "Write Object.vi"("error in (no error)"=w6558, "Object"=w6543, "Interface in"=w6555) -> ("error out"=w6557:errorcluster, "Interface out"=w6554:refnum<class "Interface.lvclass">)  [unwired: 7 in]
            n3001 = call-dynamic "Write Comments.vi"("error in (no error)"=w6557, "Comments"=w6542, "Interface in"=w6554) -> ("error out"=w6553:errorcluster, "Interface out"=w6552:refnum<class "Interface.lvclass">)  [unwired: 7 in]
            n3002 = call-dynamic "Write Observer.vi"("error in (no error)"=w6553, "Observer"=w6541, "Interface in"=w6552) -> ("error out"=w6538:errorcluster, "Interface out"=w6537:refnum<class "Interface.lvclass">)  [unwired: 7 in]
            n3003 = call-dynamic "Write Project ID.vi"("error in (no error)"=w6538, "Project ID"=w6536, "Interface in"=w6537) -> ("error out"=w6534:errorcluster, "Interface out"=w6535:refnum<class "Interface.lvclass">)  [unwired: 7 in]
            n3004 = call-dynamic "Write Interface.vi"("error in (no error)"=w6534, "Interface.lvclass"=w6535, "Channel in"=w6561) -> ("error out"=w6547:errorcluster, "Channel out"=w6548:refnum<class "Channel.lvclass">)  [unwired: 7 in]
            n3005 = call-dynamic "Read State Machine.vi"("error in (no error)"=w6547, "Device in"=w6548) -> ("error out"=w6567:errorcluster, "State Machine.lvclass"=w6571:refnum<class "State Machine.lvclass">, "Device out"=w6570:refnum<class "Channel.lvclass">)  [unwired: 7 in]
            n3006 = call-dynamic "Write State.vi"("error in (no error)"=w6567, "State"=300, "State Machine in"=w6571) -> ("error out"=w6568:errorcluster, "State Machine out"=w6572:refnum<class "State Machine.lvclass">)  [unwired: 7 in]
